vi "Set position.vi"(8 "error in":errorcluster, 10 "Stage current position":dbl[](array[numeric])) -> (0 "error out":errorcluster)   [LabVIEW 2017]
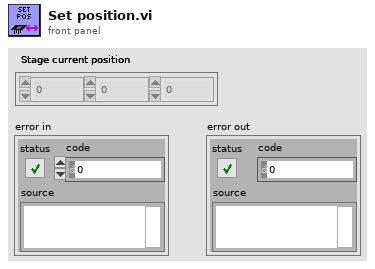
[diagram p1: front panel]
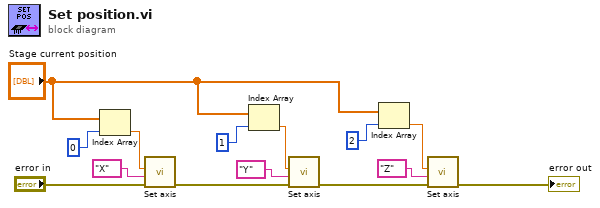
[diagram p0: block diagram]
diagram:
  n1 = Index Array(array="Stage current position", index=0) -> (element=w1:dbl)
  n2 = call "Set axis.vi"("error in"="error in", "Axis to move"="X", "New axis pos (mm)"=w1) -> ("error out"=w13:errorcluster)  [unwired: 8 in]
  n3 = Index Array(array="Stage current position", index=1) -> (element=w2:dbl)
  n4 = call "Set axis.vi"("error in"=w13, "Axis to move"="Y", "New axis pos (mm)"=w2) -> ("error out"=w12:errorcluster)  [unwired: 8 in]
  n5 = Index Array(array="Stage current position", index=2) -> (element=w3:dbl)
  n6 = call "Set axis.vi"("error in"=w12, "Axis to move"="Z", "New axis pos (mm)"=w3) -> ("error out"=→"error out":errorcluster)  [unwired: 8 in]
